vi "Camera Control.vi"(1 "i":i32) -> ()   [LabVIEW 2012]
uses:
  <vilib>/Rock Robotics/WPI/Joystick/WPI_JoystickGetSetRefNum.vi
  Robot Global Data.vi
panel:
  in  "Cam Y":dbl=50.0
  in  "Cam X":dbl=85.0
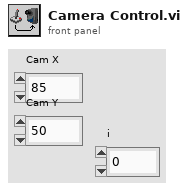
[diagram p1: front panel]
types:
  T1 = typedef "WPI_JoystickDevRef.ctl" = cluster{"Device":T2}
  T2 = typedef "WPI_JoystickDeviceEnum.ctl" = enum16{"USB 1", "USB 2", "USB 3", "USB 4", "Kinect 1", "Kinect 2"}
  T3 = typedef "WPI_JoystickButtonState.ctl" = cluster{"Button 1":bool, "Button 2":bool, "Button 3":bool, "Button 4":bool, "Button 5":bool, "Button 6":bool, "Button 7":bool, "Button 8":bool, "Button 9":bool, "Button 10":bool, "Button 11":bool, "Button 12":bool}
  T4 = cluster{"axis 1 (x)":dbl, "axis 2 (y)":dbl, "axis 3 (throttle)":dbl, "axis 4":dbl, "axis 5":dbl, "axis 6":dbl}
  T5 = typedef "WPI_ServoDeviceRef.ctl" = cluster{"DeviceStatus":errorcluster, "Digital Module":T6, "PWM Channel":T7, "DeadBand":T8}
  T6 = typedef "FPGA_TypedefDigitalModule.ctl" = enum16{"Digital Module 1", "Digital Module 2"}
  T7 = typedef "FPGA_DIOPWMChannel.ctl" = enum8{"PWM 1", "PWM 2", "PWM 3", "PWM 4", "PWM 5", "PWM 6", "PWM 7", "PWM 8", "PWM 9", "PWM 10", "Invalid"}
  T8 = typedef "WPI_PWMDeadband.ctl" = cluster{"Name":string, "maxPositivePwm":i32, "minPositivePwm":i32, "centerPwm":i32, "maxNegativePwm":i32, "minNegativePwm":i32, "angularRange":u16}
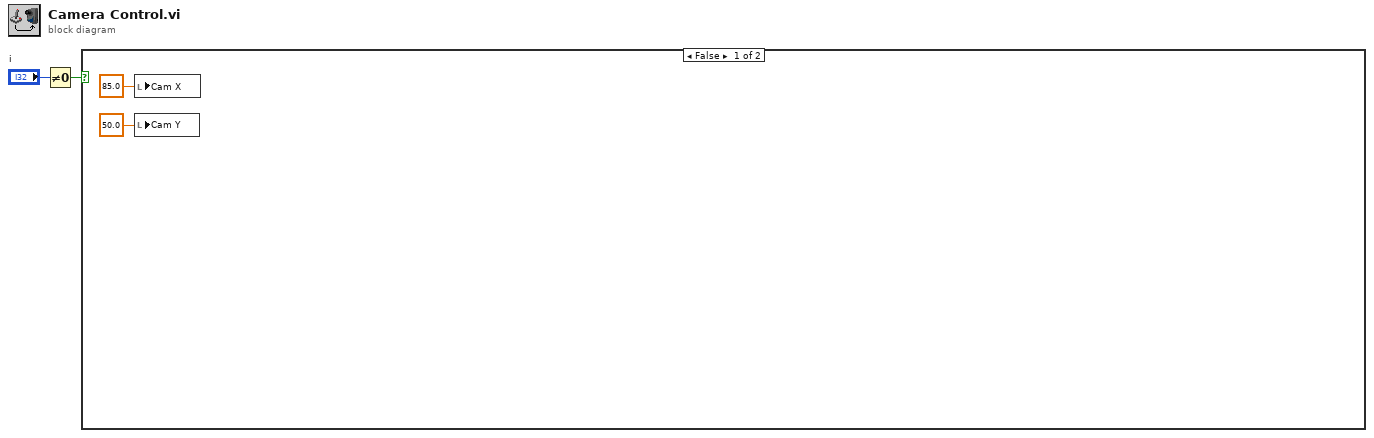
[diagram p0: block diagram]
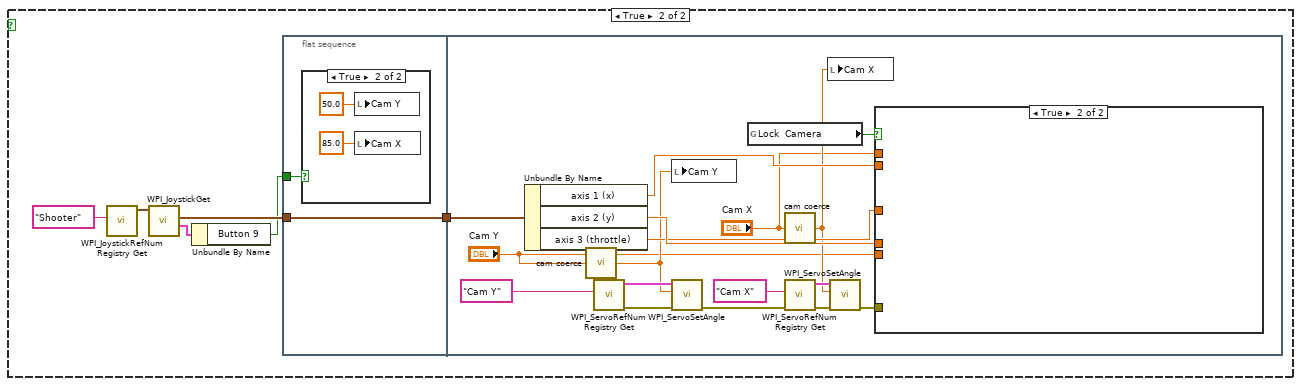
[diagram p2: hidden frame]
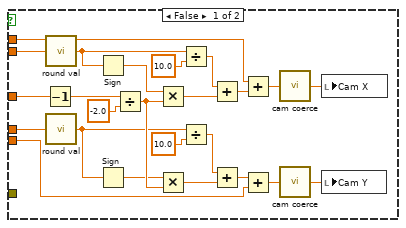
[diagram p4: hidden frame]
diagram:
  n1 = Not Equal To 0?(x="i") -> (x != 0?=w2:bool)
  n2 = case shown="False" w2 {
    frame False {
      n3 = local write "Cam X"(85.0 ("Center x")) -> ()
      n4 = local write "Cam Y"(50.0 ("Center y")) -> ()
    }
    frame True {
      n5 = call <vilib>:"WPI_JoystickRefNum Registry Get.vi"("refnum name"="Shooter") -> ("JoystickDevRef"=w9:T1)  [unwired: 1 in, 9 out]
      n6 = call <vilib>:"WPI_JoystickGet.vi"("JoystickDevRef"=w9) -> ("Buttons"=w7:T3, "Axes"=w8:T4)  [unwired: 1 in, 4 out]
      n7 = Unbundle By Name(w7) -> ("Button 9"=w5:bool)
      n8 = flat-sequence {
        tunnel: w8 -> [w12]
        tunnel: [w12] -> w6
        tunnel: w5 -> [w11]
        tunnel: w6 -> [w31]
        frame #0 {
          n9 = case shown="True" w11 {
            frame False {
            }
            frame True {
              n10 = local write "Cam Y"(50.0 ("Cam Y")) -> ()
              n11 = local write "Cam X"(85.0 ("Cam X")) -> ()
            }
          }
        }
        frame #1 {
          n12 = Unbundle By Name(w31) -> ("axis 1 (x)"=w25:dbl, "axis 2 (y)"=w24:dbl, "axis 3 (throttle)"=w23:dbl)
          n13 = call "cam coerce.vi"("x"="Cam Y") -> ("coerced(x)"=w21:dbl)
          n14 = call <vilib>:"WPI_ServoRefNum Registry Get.vi"("refnum name"="Cam Y") -> ("error out"=w16:errorcluster, "ServoDeviceRef"=w28:T5)  [unwired: 9 in]
          n15 = local write "Cam Y"(w21) -> ()
          n16 = call <vilib>:"WPI_ServoSetAngle.vi"("error in (no error)"=w16, "Angle"=w21, "ServoDeviceRef"=w28) -> ("error out"=w15:errorcluster)  [unwired: 7 in, 1 out]
          n17 = global read "Robot Global Data.vi" "Lock  Camera"() -> (w30:bool)
          n18 = call "cam coerce.vi"("x"="Cam X") -> ("coerced(x)"=w22:dbl)
          n19 = call <vilib>:"WPI_ServoRefNum Registry Get.vi"("error in (no error)"=w15, "refnum name"="Cam X") -> ("error out"=w17:errorcluster, "ServoDeviceRef"=w26:T5)  [unwired: 8 in]
          n20 = local write "Cam X"(w22) -> ()
          n21 = call <vilib>:"WPI_ServoSetAngle.vi"("error in (no error)"=w17, "Angle"=w22, "ServoDeviceRef"=w26) -> ("error out"=w18:errorcluster)  [unwired: 7 in, 1 out]
          n22 = case shown="True" w30 {
            tunnel: w25 -> [w49 _]
            tunnel: w24 -> [w48 _]
            tunnel: w23 -> [w55 _]
            tunnel: "Cam Y" -> [w37 _]
            tunnel: "Cam X" -> [w36 _]
            tunnel: w18 -> [_ _]
            frame False {
              n23 = Decrement(x=w55) -> (x-1=w54:dbl)
              n24 = call "round val.vi"("num in"=w49) -> ("num out"=w47:dbl)
              n25 = call "round val.vi"("num in"=w48) -> ("num out"=w40:dbl)
              n26 = Sign(1:w47) -> (0:w51:dbl)
              n27 = Sign(1:w40) -> (0:w50:dbl)
              n28 = Divide(x=w54, y=-2.0) -> (x/y=w52:dbl)
              n29 = Multiply(x=w51, y=w52) -> (x*y=w44:dbl)
              n30 = Multiply(x=w50, y=w52) -> (x*y=w41:dbl)
              n31 = Divide(x=w47, y=10.0) -> (x/y=w45:dbl)
              n32 = Divide(x=w40, y=10.0) -> (x/y=w42:dbl)
              n33 = Add(x=w45, y=w44) -> (x+y=w39:dbl)
              n34 = Add(x=w42, y=w41) -> (x+y=w38:dbl)
              n35 = Add(x=w36, y=w39) -> (x+y=w33:dbl)
              n36 = Add(x=w38, y=w37) -> (x+y=w35:dbl)
              n37 = call "cam coerce.vi"("x"=w33) -> ("coerced(x)"=w32:dbl)
              n38 = call "cam coerce.vi"("x"=w35) -> ("coerced(x)"=w34:dbl)
              n39 = local write "Cam X"(w32) -> ()
              n40 = local write "Cam Y"(w34) -> ()
            }
            frame True {
            }
          }
        }
      }
    }
  }
